vi "Dashboard Main.vi"() -> ()   [LabVIEW 2020]
uses:
  <vilib>/Utility/miscctls.llb/LVRowAndColumnTypeDef.ctl
  <vilib>/event_ctls.llb/eventvkey.ctl
  <vilib>/Rock Robotics/Network Tables/NT Read Numeric Array.vi
  <vilib>/Rock Robotics/WPI/Dashboard/WPI_DashboardLogging Global.vi
  <vilib>/Rock Robotics/Network Tables/NT Read Variant.vi
panel:
  out "DriveSensorData":T1
  out "NT Connection":bool
  in  "Camera Settings Right":T2={"Frame Rate"=30, "Compression"=30, "Size"=1, "DB Camera Config"=FALSE} {"Frame Rate" scale=1.0..30.0; "Compression" scale=100.0..-1.0; "Size" items=["640x480", "320x240", "160x120"]}
  in  "Camera Name Right":string(combo)="No Camera Selection"
  out "Camera Perf":string
  in  "Camera Settings":T2={"Frame Rate"=30, "Compression"=30, "Size"=1, "DB Camera Config"=FALSE} {"Frame Rate" scale=1.0..30.0; "Compression" scale=100.0..-1.0; "Size" items=["640x480", "320x240", "160x120"]}
  in  "TCP":refnum<k5>
  in  "Rec Mode":enum32{"Stop", "Record", "Playback"}(radio)
  out "Robot IP":string
  out "Image Message":string="Timeout in Camera Communications"
  in  "Dashboard Tab":T3(tab)
  out "Mode":T4(ring)=enum."Auto Disabled"
  out "Right Camera Perf":cluster{"Bandwidth (Mbps)":dbl, "FPS":dbl}
  in  "StartingPosition":dbl
  in  "AutoFileName (No .txt)":string
  in  "WaitAtStartOfAuto (Seconds)":dbl
  out "AutoFilesOnRobot":string[](array[string])
  out "Camera Image Right":T5(plugin-control)
  in  "DB/String 9":string
  in  "DB/String 8":string
  in  "DB/String 7":string
  in  "DB/String 6":string
  in  "DB/String 5":string
  in  "DB/String 4":string
  in  "DB/String 3":string
  in  "DB/String 2":string
  in  "DB/String 1":string
  in  "DB/String 0":string
  in  "DB/Slider 0":dbl(slide) scale=0.0..5.0
  in  "DB/Slider 1":dbl(slide) scale=0.0..5.0
  in  "DB/Slider 2":dbl(slide) scale=0.0..5.0
  in  "DB/Slider 3":dbl(slide) scale=0.0..5.0
  out "DB/LED 3":bool
  out "DB/LED 2":bool
  out "DB/LED 1":bool
  out "DB/LED 0":bool
  in  "DB/Button 3":bool
  in  "DB/Button 2":bool
  in  "DB/Button 1":bool
  in  "DB/Button 0":bool caption="New Name"
  in  "Test Slider":dbl(slide) scale=0.0..100.0 scale format="%#_3g"
  in  "On/Off":bool caption="Solenoid"
  in  "Test Name":u16(ring) items=["Select the test to run..."]
  in  "Test Tree":string(tree)
  in  "Motor":cluster{"Value":dbl, "Enable":bool} {"Value" scale=-1.0..1.0 scale format="%#_3g"}
  out "Progress":T6 {"Test Progress" scale=0.0..100.0}
  in  "Rev/Fwd":cluster{"Forward":bool, "Reverse":bool}
  in  "Test Ring":u16(ring) items=["Monochrome", "Color"]
  out "Cmd Status":string
  in  "Execute Command":bool
  in  "Command Params":string[][](table)
  in  "Command Selection":i32(listbox)
  in  "CheckList":i32(listbox)
  out "Tree":string(tree)
  out "Camera Image":T5(plugin-control)
  in  "Camera Name":string(combo)="No Camera Selection"
  # "HW"
  # "HW"
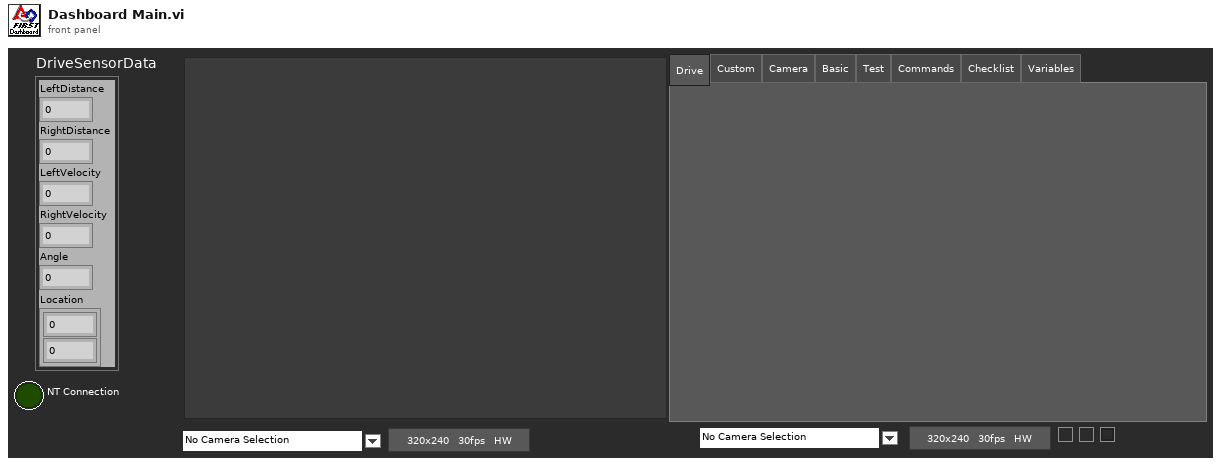
[diagram p1: front panel]
types:
  T1 = cluster{"LeftDistance":dbl, "RightDistance":dbl, "LeftVelocity":dbl, "RightVelocity":dbl, "Angle":dbl, "Location":cluster{dbl, dbl}}
  T2 = cluster{"Frame Rate":i32, "Compression":i32, "Size":u16, "DB Camera Config":bool}
  T3 = enum32{"Drive", "Custom", "Camera", "Basic", "Test", "Commands", "Checklist", "Variables"}
  T4 = enum8{"Tele-Op Disabled", "Tele-Op Enabled", "Auto Disabled", "Auto Enabled", "Test Disabled", "Test Enabled", "Disconnected", "No Code", "E-Stop"}
  T5 = typedef "IMAQ Image.ctl" = refnum<image>
  T6 = cluster{"Test Progress":u8, "Test Progress Text":string}
  T7 = cluster{"Save Path":path, "Interval (s)":dbl, "Keep":i32}
  T8 = enum32{"Drive", "Camera", "Basic", "Custom", "Test", "Commands", "Checklist", "Variables"}
  T9 = typedef "Image Type" = u32
  T10 = cluster{"IDs":cluster{"RPC field ID":u16, "Unique ID":u16}, "String":string}
  T11 = cluster{"Error Strings":string, "Disable Counts":cluster{u16, u16}, "Rail Faults":cluster{u16, u16, u16}, "Robot IP":string, "DB Mode":u8, "Event Info":cluster{"Name":string, "Type":u8, "Number":u16, "Replay":u8}}
  T12 = cluster{"Storage":cluster{"Disk Free":u64, "RAM Block":u32, "RAM free":u32}, "CPU Utilization":cluster{"CPU % ISR":sgl, "CPU % Time Crit":sgl, "CPU % Timed Str":sgl, "CPU % High":sgl, "CPU % Above":sgl, "CPU % Normal":sgl, "CPU % Low":sgl}, "CAN":cluster{"% Bus Utilization":sgl, "Bus Off Cnt":u32, "TX_FIFO Full Cnt":u32, "Receive Error Cnt":u8, "Transmit Error Cnt":u8}, "HID":cluster{"HID Outputs":u32, "Rumble Low":u16, "Rumble High":u16}[]}
  T13 = cluster{"Status bits":cluster{"Test Mode":bool, "Autonomous":bool, "Enabled":bool, "Code Start":bool, "Brownout":bool, "Reserved 2":bool, "Reserved 3":bool, "E-Stop":bool}, "Code Trace":cluster{"Disabled":bool, "TeleOp":bool, "Auto":bool, "Test":bool}, "Controller Type":enum16{"unknown", "cRIO", "roboRio"}, "Code?":enum16{"unknown", "noCode", "code"}, "Battery V":dbl}
  T14 = cluster{"Control Bits":cluster{"TestMode":bool, "Autonomous":bool, "Enabled":bool, "FMS Present":bool, bool, bool, bool, "E-Stop":bool}, "Team Station ":u8, "Countdown":sgl, "Joystick Values":cluster{"Axes":dbl[], "Buttons":bool[], "POVs":i16[]}[]}
  T15 = cluster{"Axes":dbl[], "Buttons":bool[], "POVs":i16[]}[]
  T16 = cluster{"Axes":dbl[], "Buttons":bool[], "POVs":i16[]}
  T17 = cluster{"Global Rectangle":i32[], "Contours":cluster{"Contour Type":u32, "ROI Type":u32, "Points":i32[]}[]}
  T18 = cluster{"Camera Name":string, string, "Saved DB Images Info":cluster{"Save Path":path, "Interval (s)":dbl, "Keep":i32}}
  T19 = cluster{"Camera Name Right":string, string, "Saved DB Images Info":cluster{"Save Path":path, "Interval (s)":dbl, "Keep":i32}}
  T20 = cluster{"Operation":enum16{"Update", "Clear"}, "Color Box":u32}[]
  T21 = typedef "eventvkey.ctl" = enum16{"ASCII", "Enter", "Return", "Shift", "Ctrl", "Alt", "Cmd", "Opt", "Caps", "NumLock", "Clear", "Break", "Up", "Down", "Left", "Right", "Insert", "Delete", "Home", "End", "PageUp", "PageDown", "Escape", "Help", "Pause", "ScrollLock", "F1", "F2", "F3", "F4", "F5", "F6", "F7", "F8", "F9", "F10", "F11", "F12", "F13", "F14", "F15", "F16", "F17", "F18", "F19", "F20", "F21", "F22", "F23", "F24", "Play", "VolumeUp", "VolumeDown", "Mute", "Two Byte Char"}
  T22 = cluster{"Image Size":bool, "Image Type":bool, "Pixel Value":bool, "ROI Information":bool, "Zoom Factor":bool}
  T23 = cluster{"Operation":enum16{"Update", "Clear"}, "Color Box":u32}
  T24 = typedef "LVRowAndColumnTypeDef.ctl" = cluster{"Row":i32, "Column":i32}
  T25 = cluster{"Shift":bool, "Ctrl":bool, "Alt":bool, "Cmd":bool, "Opt":bool}
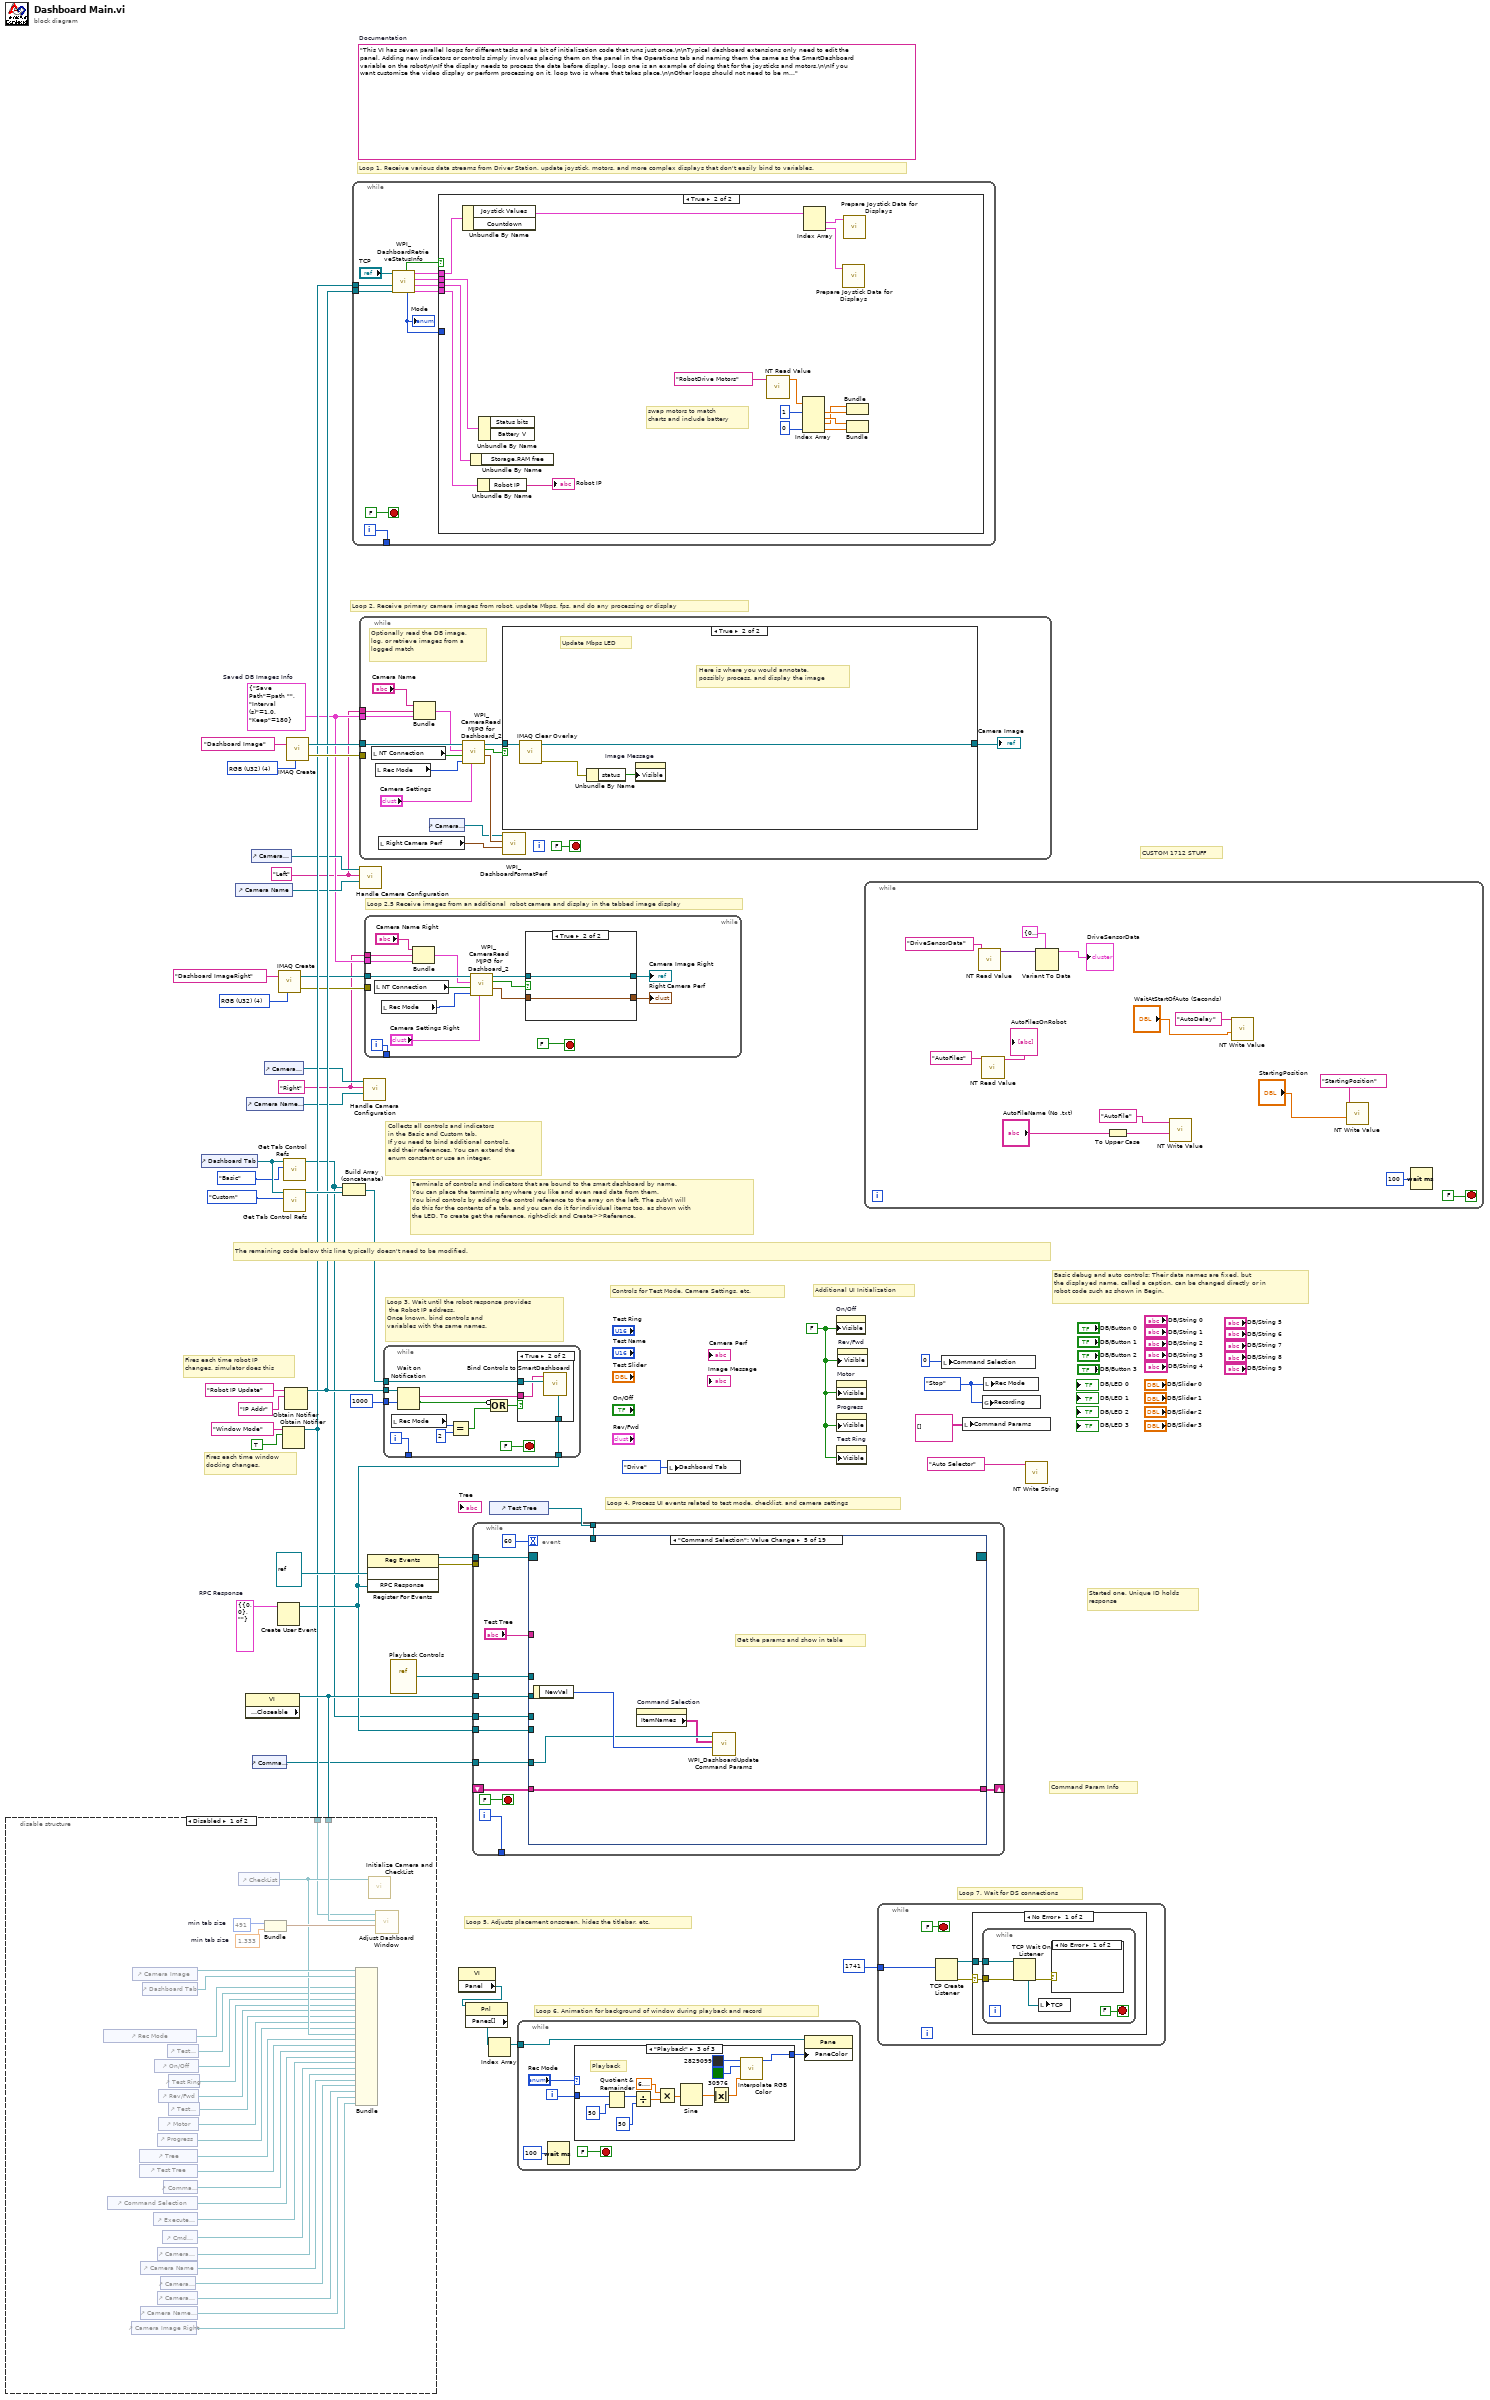
[diagram p0: block diagram]
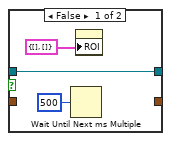
[diagram p3: hidden frame]
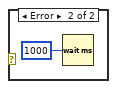
[diagram p4: hidden frame]
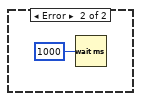
[diagram p5: hidden frame]
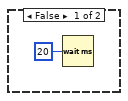
[diagram p6: hidden frame]
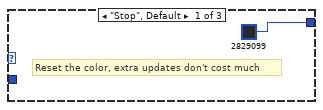
[diagram p7: hidden frame]
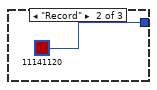
[diagram p8: hidden frame]
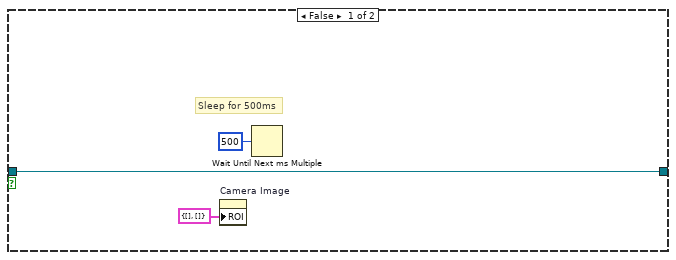
[diagram p10: hidden frame]
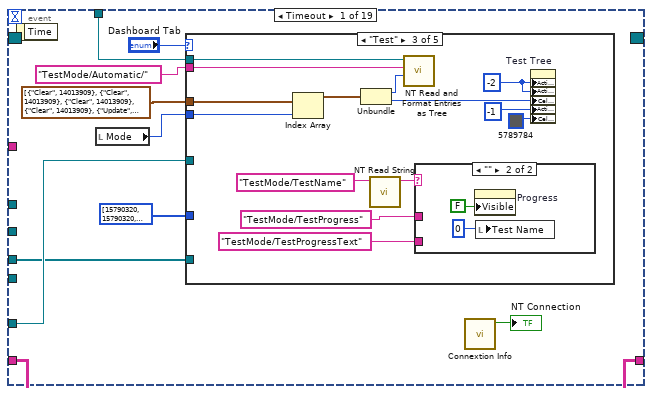
[diagram p11: hidden frame]
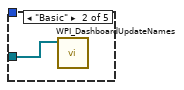
[diagram p13: hidden frame]
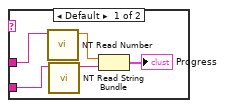
[diagram p14: hidden frame]
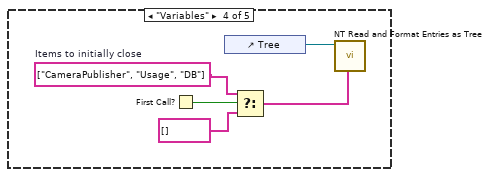
[diagram p15: hidden frame]
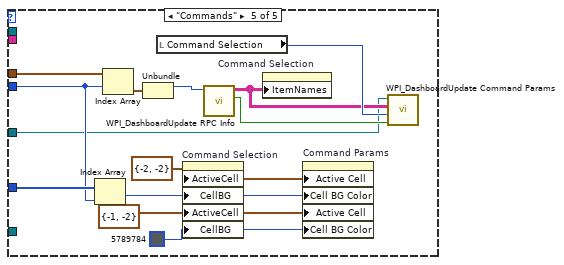
[diagram p16: hidden frame]
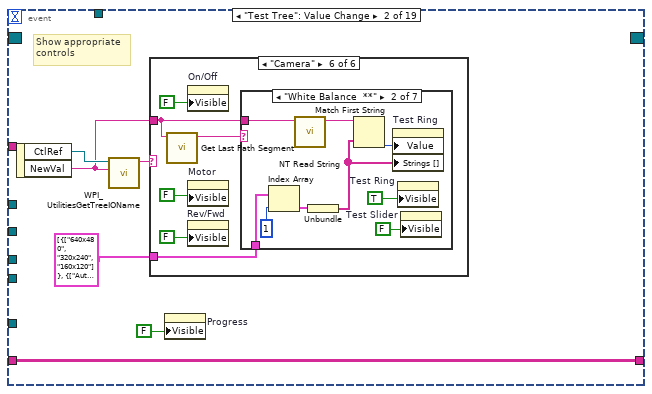
[diagram p17: hidden frame]
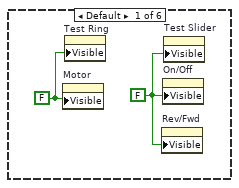
[diagram p18: hidden frame]
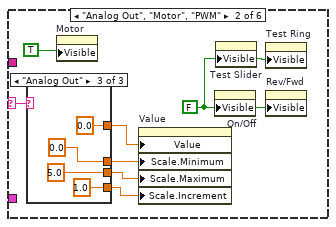
[diagram p19: hidden frame]
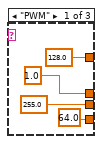
[diagram p20: hidden frame]
diagram:
  w4 = T7 {"Save Path"=path "", "Interval (s)"=1.0, "Keep"=180}  # Saved DB Images Info
  w3 = "Right"
  w2 = "Left"
  w11 = T9 4 items=["Grayscale (U8)", "Grayscale (I16)", "Grayscale (SGL)", "Complex (CSG)", "RGB (U32)", "HSL (U32)", "RGB (U64)"] ("Image Type")
  w21 = T10 {"IDs"={"RPC field ID"=0, "Unique ID"=0}, "String"=""}  # RPC Response
  w30 = enum32{"Stop", "Record", "Playback"}."Stop" ("Rec Mode")
  w25 = FALSE ("Visible")
  (unwired) "This VI has seven parallel loops for different tasks and a bit of initialization code that runs just once.\n\nTypical dashboard extensions only need to edit the panel. Adding new indicators or controls simply involves placing them on the panel in the Operations tab and naming them the same as the SmartDashboard variable on the robot\n\nIf the display needs to process the data before display, loop one is an example of doing that for the joysticks and motors.\n\nIf you want customize the video display or perform processing on it, loop two is where that takes place.\n\nOther loops should not need to be modified. They are pretty standard, and document the task they perform."  # Documentation
  w47 = T9 4 items=["Grayscale (U8)", "Grayscale (I16)", "Grayscale (SGL)", "Complex (CSG)", "RGB (U32)", "HSL (U32)", "RGB (U64)"] ("Image Type")
  # "CUSTOM 1712 STUFF"
  # "Loop 2.5 Receive images from an additional  robot camera and display in the tabbed image display"
  # "Command Param Info"
  # "Started one, Unique ID holds\nresponse"
  # "Loop 7. Wait for DS connections"
  # "Basic debug and auto controls: Their data names are fixed, but\nthe displayed name, called a caption, can be changed directly or in\nrobot code such as shown in Begin."
  # "Controls for Test Mode, Camera Settings, etc."
  # "Additional UI Initialization"
  # "Loop 6. Animation for background of window during playback and record"
  # "Fires each time robot IP\nchanges, simulator does this"
  # "Fires each time window\ndocking changes."
  # "Collects all controls and indicators\nin the Basic and Custom tab.\nIf you need to bind additional controls,\nadd their references. You can extend the\nenum constant or use an integer."
  # "The remaining code below this line typically doesn't need to be modified."
  # "Loop 4. Process UI events related to test mode, checklist, and camera settings"
  # "Terminals of controls and indicators that are bound to the smart dashboard by name.\nYou can place the terminals anywhere you like and even read data from them.\nYou bind controls by adding the control reference to the array on the left. The subVI will\ndo this for the contents of a tab, and you can do it for individual items too, as shown with\nthe LED. To create get the reference, right-click and Create>>Reference."
  # "Loop 3. Wait until the robot response provides\n the Robot IP address.\nOnce known, bind controls and\nvariables with the same names."
  # "Loop 5. Adjusts placement onscreen, hides the titlebar, etc."
  # "Loop 1. Receive various data streams from Driver Station, update joystick, motors, and more complex displays that don't easily bind to variables."
  # "Loop 2. Receive primary camera images from robot, update Mbps, fps, and do any processing or display"
  n1 = control-ref of="Dashboard Tab"() -> (w28:refnum<vi>)
  n2 = control-ref of="Camera Name"() -> (w15:refnum<vi>)
  n3 = property class="VI" props=["Front Panel.Closeable"]() -> (reference out=w29:refnum<vi>)  [unwired: 2 in, 2 out]
  n4 = control-ref of="Camera Name Right"() -> (w7:refnum<vi>)
  n5 = control-ref of="Camera Settings"() -> (w16:refnum<vi>)
  n6 = control-ref of="Command Params"() -> (w17:refnum<vi>)
  n7 = control-ref of="Camera Settings Right"() -> (w8:refnum<vi>)
  n8 = Create User Event(user event datatype=w21) -> (user event=w18:refnum<user-event>)  [unwired: 1 in, 1 out]
  n9 = call "IMAQ Create"("Image Name"="Dashboard ImageRight", "Image Type"=w11) -> ("New Image"=w10:T5, "error out"=w9:errorcluster)  [unwired: 2 in, 1 out]
  n10 = Obtain Notifier(name (unnamed)="Window Mode", notification data type=TRUE) -> (notifier out=w23:refnum<notifier>)  [unwired: 2 in, 2 out]
  n11 = disable-structure shown="Disabled" {
    disable-tunnel: w29 -> [w75 _]
    disable-tunnel: w23 -> [w58 _]
    frame Disabled {
      w72 = 491  # min tab size
      w71 = 1.333  # min tab size
      n12 = control-ref of="Rec Mode"() -> (w64:refnum<vi>)
      n13 = control-ref of="Command Selection"() -> (w55:refnum<vi>)
      n14 = control-ref of="Camera Image Right"() -> (w48:refnum<vi>)
      n15 = control-ref of="Camera Image"() -> (w74:refnum<vi>)
      n16 = control-ref of="Tree"() -> (w68:refnum<vi>)
      n17 = control-ref of="Test Tree"() -> (w67:refnum<vi>)
      n18 = control-ref of="Camera Name"() -> (w52:refnum<vi>)
      n19 = control-ref of="Camera Name Right"() -> (w49:refnum<vi>)
      n20 = control-ref of="Dashboard Tab"() -> (w73:refnum<vi>)
      n21 = control-ref of="Execute Command"() -> (w56:refnum<vi>)
      n22 = control-ref of="On/Off"() -> (w62:refnum<vi>)
      n23 = control-ref of="Progress"() -> (w59:refnum<vi>)
      n24 = control-ref of="Camera Settings"() -> (w53:refnum<vi>)
      n25 = control-ref of="Camera Settings Right"() -> (w50:refnum<vi>)
      n26 = control-ref of="Rev/Fwd"() -> (w60:refnum<vi>)
      n27 = control-ref of="Motor"() -> (w65:refnum<vi>)
      n28 = control-ref of="Camera Perf"() -> (w51:refnum<vi>)
      n29 = control-ref of="Cmd Status"() -> (w54:refnum<vi>)
      n30 = control-ref of="Command Params"() -> (w57:refnum<vi>)
      n31 = control-ref of="Test Slider"() -> (w63:refnum<vi>)
      n32 = control-ref of="Test Ring"() -> (w61:refnum<vi>)
      n33 = control-ref of="Test Name"() -> (w66:refnum<vi>)
      n34 = control-ref of="CheckList"() -> (w69:refnum<vi>)
      n35 = Bundle("min tab size"=w72, "min tab size"=w71) -> (w70:cluster{"min tab size":i32, "min tab size":dbl})  [unwired: 1 in]
      n36 = Bundle("Camera Image"=w74, "Dashboard Tab"=w73, "Rec Mode"=w64, "Test Slider"=w63, "On/Off"=w62, "Test Ring"=w61, "Rev/Fwd"=w60, "Test Name"=w66, "Motor"=w65, "Progress"=w59, "CheckList"=w69, "Tree"=w68, "Test Tree"=w67, "Command Params"=w57, "Command Selection"=w55, "Execute Command"=w56, "Cmd Status"=w54, "Camera Settings"=w53, "Camera Name"=w52, "Camera Perf"=w51, "Camera Settings Right"=w50, "Camera Name Right"=w49, "Camera Image Right"=w48) -> ()  [unwired: 2 in, 1 out]
      n37 = call "Initialize Camera and CheckList.vi"("ListBox in"=w69) -> ()  [unwired: 11 in]
      n38 = call "Adjust Dashboard Window.vi"("Size Constraints"=w70, "VI"=w75, "WIn Mode"=w58) -> ()  [unwired: 9 in]
    }
    frame Enabled {
    }
  }
  n39 = call <vilib>:"Get Tab Control Refs.vi"("Page Index"=T8."Basic" ("Dashboard Tab"), "TabControl in"=w28) -> ("ControlsOnPage"=w14:refnum<vi>[])  [unwired: 9 in]
  n40 = call <vilib>:"Get Tab Control Refs.vi"("Page Index"=T8."Custom" ("Dashboard Tab"), "TabControl in"=w28) -> ("ControlsOnPage"=w27:refnum<vi>[])  [unwired: 9 in]
  n41 = Obtain Notifier(name (unnamed)="Robot IP Update", notification data type="IP Addr" ("name (unnamed)")) -> (notifier out=w24:refnum<notifier>)  [unwired: 2 in, 2 out]
  n42 = call "IMAQ Create"("Image Name"="Dashboard Image", "Image Type"=w47) -> ("New Image"=w45:T5, "error out"=w44:errorcluster)  [unwired: 2 in, 1 out]
  n43 = Build Array (concatenate)(w14, w27) -> (w26:refnum<vi>[])
  n44 = while {
    tunnel: [w85] -> _
    tunnel: w24 -> [w79]
    tunnel: w23 -> [w76]
    i -> [w85]
    stop <- FALSE stop-if-true
    n45 = call <vilib>:"WPI_DashboardRetrieveStatusInfo.vi"("Binding Refnum"=w79, "Window Mode Notifier"=w76, "TCP Cnx"="TCP") -> ("Power and Errors"=w80:T11, "Robot Metrics"=w83:T12, "Status Info"=w84:T13, "Control Info"=w81:T14, "Robot Mode"=w78:T4, "Process?"=w82:bool)  [unwired: 3 in]
    "Mode" <- w78
    n46 = case shown="True" w82 {
      tunnel: w84 -> [_ w103]
      tunnel: w83 -> [_ w102]
      tunnel: w81 -> [_ w101]
      tunnel: w80 -> [_ w100]
      tunnel: w78 -> [_ _]
      frame False {
        n47 = Wait (ms)(milliseconds to wait=u32 20) -> ()  [unwired: 1 out]
      }
      frame True {
        # "swap motors to match\ncharts and include battery"
        n48 = Unbundle By Name(w101) -> ("Joystick Values"=w93:T15)  [unwired: 1 out]
        n49 = Unbundle By Name(w102) -> ()  [unwired: 1 out]
        n50 = Unbundle By Name(w100) -> ("Robot IP"=→"Robot IP":string)
        n51 = Unbundle By Name(w103) -> ()  [unwired: 2 out]
        n52 = call-poly <vilib>:"NT Read Value.vi"("Name"="RobotDrive Motors") -> ("Numeric Array"=w89:dbl[])  [unwired: 9 in, 1 out]
        n53 = Index Array(array=w89, index #1=1, index #4=0) -> (element #1=w95:dbl, element #2=w96:dbl, element #3=w94:dbl, element #4=w99:dbl)  [unwired: 2 in]
        n54 = Index Array(array=w93) -> (element #1=w92:T16, element #2=w91:T16)  [unwired: 2 in]
        n55 = call "Prepare Joystick Data for Displays.vi"("Joystick Values"=w91) -> ()  [unwired: 8 in, 3 out]
        n56 = call "Prepare Joystick Data for Displays.vi"("Joystick Values"=w92) -> ()  [unwired: 8 in, 3 out]
        n57 = Bundle("Numeric"=w94, "Numeric"=w95) -> ()  [unwired: 1 in, 1 out]
        n58 = Bundle("Numeric"=w96, "Numeric"=w99) -> ()  [unwired: 1 in, 1 out]
      }
    }
  }
  n59 = call "Handle Camera Configuration.vi"("CameraNameRef"=w15, "Display Name"=w2, "ClusterRef"=w16) -> ()  [unwired: 9 in]
  n60 = while {
    tunnel: w45 -> [w117]
    tunnel: w44 -> [_]
    tunnel: w4 -> [w110]
    tunnel: w2 -> [w107]
    stop <- FALSE stop-if-true
    # "Optionally read the DB image,\nlog, or retrieve images from a\nlogged match"
    n61 = local read "NT Connection"() -> (w111:bool)
    n62 = local read "Rec Mode"() -> (w114:enum32{"Stop", "Record", "Playback"})
    n63 = local read "Right Camera Perf"() -> (w105:cluster{"Bandwidth (Mbps)":dbl, "FPS":dbl})
    n64 = Bundle("Camera Name"="Camera Name", w107, "Saved DB Images Info"=w110) -> (w109:T18)  [unwired: 1 in]
    n65 = control-ref of="Camera Perf"() -> (w104:refnum<vi>)
    n66 = call <vilib>:"WPI_CameraRead MJPG for Dashboard_2.vi"("Camera Settings"="Camera Settings", "Rec Mode"=w114, "NT Connection"=w111, "Capture Info"=w109, "Image in"=w117) -> ("perf info"=w106:cluster{"Bandwidth (Mbps)":dbl, "fps":dbl}, "Active"=w115:bool, "Image\\ out"=w116:T5)  [unwired: 4 in]
    n67 = case shown="True" w115 {
      tunnel: w116 -> [w120 w123]
      tunnel: [w120 w122] -> w112
      frame False {
        # "Sleep for 500ms"
        n68 = property on="Camera Image" class="ImageControl"("ROI"=T17 {"Global Rectangle"=[], "Contours"=[]}) -> ()  [unwired: 2 in, 2 out]
        n69 = Wait Until Next ms Multiple(millisecond multiple=u32 500) -> ()  [unwired: 1 out]
      }
      frame True {
        # "Here is where you would annotate,\npossibly process, and display the image"
        # "Update Mbps LED"
        n70 = call "IMAQ Clear Overlay"("Image"=w123) -> ("error out"=w124:errorcluster, "Image Out"=w122:T5)  [unwired: 2 in, 7 out]
        n71 = Unbundle By Name(w124) -> ("status"=w125:bool)
        n72 = property on="Image Message" class="Str"("Visible"=w125) -> ()  [unwired: 2 in, 2 out]
      }
    }
    "Camera Image" <- w112
    n73 = call <vilib>:"WPI_DashboardFormatPerf.vi"("Right Camera Perf"=w105, "Performance"=w106, "String in"=w104) -> ()  [unwired: 9 in]
  }
  n74 = call "Handle Camera Configuration.vi"("CameraNameRef"=w7, "Display Name"=w3, "ClusterRef"=w8) -> ()  [unwired: 9 in]
  n75 = while {
    tunnel: w10 -> [w140]
    tunnel: w9 -> [_]
    tunnel: [w135] -> _
    tunnel: w4 -> [w131]
    tunnel: w3 -> [w128]
    i -> [w135]
    stop <- FALSE stop-if-true
    n76 = local read "NT Connection"() -> (w132:bool)
    n77 = local read "Rec Mode"() -> (w139:enum32{"Stop", "Record", "Playback"})
    n78 = Bundle("Camera Name Right"="Camera Name Right", w128, "Saved DB Images Info"=w131) -> (w130:T19)  [unwired: 1 in]
    n79 = call <vilib>:"WPI_CameraRead MJPG for Dashboard_2.vi"("Camera Settings"="Camera Settings Right", "Rec Mode"=w139, "NT Connection"=w132, "Capture Info"=w130, "Image in"=w140) -> ("perf info"=w126:cluster{"Bandwidth (Mbps)":dbl, "fps":dbl}, "Active"=w134:bool, "Image\\ out"=w137:T5)  [unwired: 4 in]
    n80 = case shown="True" w134 {
      tunnel: w137 -> [w142 w145]
      tunnel: [w142 w145] -> w133
      tunnel: [_ w144] -> w127
      tunnel: w126 -> [_ w144]
      frame False {
        n81 = Wait Until Next ms Multiple(millisecond multiple=u32 500) -> ()  [unwired: 1 out]
        n82 = property on="Camera Image Right" class="ImageControl"("ROI"=T17 {"Global Rectangle"=[], "Contours"=[]}) -> ()  [unwired: 2 in, 2 out]
      }
      frame True {
      }
    }
    "Camera Image Right" <- w133
    "Right Camera Perf" <- w127
  }
  n83 = register-events(refnum<vi> refnum, w18) -> (reference out=w34:refnum<event-registration>, error out=w33:errorcluster)  [unwired: 2 in]
  n84 = while {
    tunnel: w26 -> [w157]
    tunnel: w24 -> [w155]
    tunnel: [w153] -> _
    tunnel: u32 1000 ("milliseconds to wait") -> [w152]
    tunnel: w18 -> [w146]
    i -> [w153]
    stop <- FALSE stop-if-true
    n85 = local read "Rec Mode"() -> (w148:enum32{"Stop", "Record", "Playback"})
    n86 = Wait on Notification(notifier=w155, timeout in ms (-1)=w152) -> (notification=w154:string, timed out?=w150:bool)  [unwired: 2 in, 2 out]
    n87 = Equal?(x=w148, y=u16 2 ("Rec Mode")) -> (x = y?=w149:bool)
    n88 = Compound Arithmetic op=OR(invert w150, w149) -> (w151:bool)
    n89 = case shown="True" w151 {
      tunnel: w157 -> [_ w160]
      tunnel: w154 -> [_ w159]
      tunnel: w146 -> [_ w158]
      frame False {
      }
      frame True {
        n90 = call <vilib>:"Bind Controls to SmartDashboard.vi"("RPC ref"=w158, "Bound Control Refs"=w160, "Server IP Address"=w159) -> ()  [unwired: 9 in]
      }
    }
  }
  n91 = vi-ref "Playback Controls.vi"() -> (w35:refnum<vi>)
  n92 = property class="VI"() -> ("Panel"=w37:refnum<vi>)  [unwired: 2 in, 2 out]
  n93 = property class="Pnl"(reference=w37) -> ("Panes[]"=w38:refnum<vi>[])  [unwired: 1 in, 2 out]
  n94 = Index Array(array=w38) -> (element=w36:refnum<vi>)  [unwired: 1 in]
  n95 = control-ref of="Test Tree"() -> (w39:refnum<vi>)
  n96 = while {
    tunnel: [w170] -> _
    tunnel: w39 -> [w169]
    tunnel: w35 -> [w168]
    tunnel: w34 -> [w167]
    tunnel: w33 -> [_]
    tunnel: w29 -> [w166]
    tunnel: w18 -> [w165]
    tunnel: w17 -> [w164]
    shift-right: [w163] -> _
    shift-left: _ -> [w162]
    tunnel: w14 -> [w161]
    i -> [w170]
    stop <- FALSE stop-if-true
    n97 = event shown="[4] \"Command Selection\": Value Change" {
      selector: w167 -> [_ _ _ _ _ _ _ _ _ _ _ _ _ _ _ _ _ _ _]
      dyn-events: [_ _ _ _ _ _ _ _ _ _ _ _ _ _ w424 _ _ _ _] -> _
      timeout: u32 60 ("milliseconds to wait") -> [_ _ _ _ _ _ _ _ _ _ _ _ _ _ _ _ _ _ _]
      tunnel: w169 -> [w182 _ _ _ _ _ _ _ _ _ _ _ _ _ _ _ _ _ _]
      tunnel: "Test Tree" -> [_ _ _ _ _ _ _ _ _ w391 w399 w401 w405 w413 _ _ _ _ _]
      tunnel: w168 -> [_ _ _ _ _ _ _ _ _ _ _ _ _ _ w426 _ w444 _ _]
      tunnel: w166 -> [_ _ _ _ _ _ _ _ _ _ _ _ _ _ w422 _ _ _ _]
      tunnel: w165 -> [_ _ _ _ _ _ _ _ _ _ _ _ _ _ w420 _ _ _ _]
      tunnel: w164 -> [w177 _ _ _ w342 _ _ _ _ _ _ _ _ _ _ _ _ _ _]
      tunnel: [w176 w225 w327 w332 w340 w349 w359 w366 w378 w390 w397 w400 w404 w412 w419 w439 w441 w445 w458] -> w163
      tunnel: w162 -> [w176 w225 w327 w332 w340 _ _ w366 w378 w390 w397 w400 w404 w412 w419 w439 w441 w445 w458]
      tunnel: w161 -> [w174 _ _ _ _ _ _ _ _ _ _ _ _ _ _ _ _ _ _]
      event Timeout {
        n98 = event-data() -> ()  [unwired: 1 in, 1 out]
        n99 = local read "Mode"() -> (w179:T4)
        n100 = case shown="\"Test\"" "Dashboard Tab" {
          tunnel: w182 -> [_ _ w198 _ _]
          tunnel: "TestMode/Automatic/" ("Name Pattern") -> [_ _ w197 _ _]
          tunnel: T20 [{"Operation"=enum."Clear", "Color Box"=14013909}, {"Operation"=enum."Clear", "Color Box"=14013909}, {"Operation"=enum."Clear", "Color Box"=14013909}, {"Operation"=enum."Clear", "Color Box"=14013909}, {"Operation"=enum."Update", "Color Box"=14013909}, {"Operation"=enum."Update", "Color Box"=16777215}, {"Operation"=enum."Clear", "Color Box"=14013909}, {"Operation"=enum."Clear", "Color Box"=14013909}, {"Operation"=enum."Clear", "Color Box"=14013909}] -> [_ _ w190 _ w218]
          tunnel: w179 -> [_ _ w189 _ w217]
          tunnel: u32[] [15790320, 15790320, 15790320, 15790320, 16777215, 16777215, 15790320, 15790320, 15790320] -> [_ _ _ _ w223]
          tunnel: w177 -> [_ _ _ _ w211]
          tunnel: w174 -> [_ w184 _ _ _]
          frame "Custom", Default {
          }
          frame "Basic" {
            n101 = call <vilib>:"WPI_DashboardUpdateNames.vi"("Controls on Tab"=w184) -> ()  [unwired: 11 in]
          }
          frame "Test" {
            w196 = -2 ("Active Item:Row Number")
            n102 = Index Array(array=w190, index=w189) -> (element=w191:T23)
            n103 = Unbundle(w191) -> ("Operation"=w192:enum16{"Update", "Clear"}, "Color Box"=w193:u32)
            n104 = call <vilib>:"NT Read String.vi"("Name"="TestMode/TestName") -> ("String"=w187:string)  [unwired: 9 in, 1 out]
            n105 = call <vilib>:"NT Read and Format Entries as Tree.vi"("Operation"=w192, "Name Pattern"=w197, "Tree Refnum"=w198) -> ()  [unwired: 7 in, 2 out]
            n106 = case shown="\"\"" w187 {
              tunnel: "TestMode/TestProgress" ("Name") -> [w200 _]
              tunnel: "TestMode/TestProgressText" ("Name") -> [w199 _]
              frame Default {
                n107 = call <vilib>:"NT Read Number.vi"("Name"=w200) -> ("Numeric"=w201:dbl)  [unwired: 9 in, 1 out]
                n108 = call <vilib>:"NT Read String.vi"("Name"=w199) -> ("String"=w202:string)  [unwired: 9 in, 1 out]
                n109 = Bundle("Numeric"=w201, "String"=w202) -> (→"Progress":cluster{"Numeric":dbl, "String":string})  [unwired: 1 in]
              }
              frame "" {
                n110 = property on="Progress" class="Clust (strict)"("Visible"=FALSE) -> ()  [unwired: 2 in, 2 out]
                n111 = local write "Test Name"(u16 0) -> ()
              }
            }
            n112 = property on="Test Tree" class="Tree (strict)"("Active Item Row Number"=w196, "ActiveColNum"=w196, "CellBG"=w193, "Active Item Row Number"=-1 ("Active Item:Row Number"), "CellBG"=u32 5789784 ("Color Box")) -> ()  [unwired: 2 in, 2 out]
          }
          frame "Variables" {
            w208 = string[] ["CameraPublisher", "Usage", "DB"]  # Items to initially close
            n113 = First Call?() -> (First Call?: T/F=w209:bool)
            n114 = control-ref of="Tree"() -> (w210:refnum<vi>)
            n115 = Select(t=w208, s=w209, f=string[] []) -> (s? t:f=w206:string[])
            n116 = call <vilib>:"NT Read and Format Entries as Tree.vi"("Tags to  Close"=w206, "Tree Refnum"=w210) -> ()  [unwired: 8 in, 2 out]
          }
          frame "Commands" {
            w219 = u32 5789784 ("Color Box")
            w220 = T24 {"Row"=-1, "Column"=-2} ("Active Cell:Active Cell")
            w222 = T24 {"Row"=-2, "Column"=-2} ("Active Cell:Active Cell")
            n117 = Index Array(array=w223, index=w217) -> (element=w221:u32)
            n118 = Index Array(array=w218, index=w217) -> (element=w216:T23)
            n119 = Unbundle(w216) -> ("Operation"=w215:enum16{"Update", "Clear"})  [unwired: 1 out]
            n120 = local read "Command Selection"() -> (w214:i32)
            n121 = property on="Command Selection" class="MCListbox (strict)"("ActiveCell"=w222, "CellBG"=w221, "ActiveCell"=w220, "CellBG"=w219) -> ()  [unwired: 2 in, 2 out]
            n122 = call <vilib>:"WPI_DashboardUpdate RPC Info.vi"("Operation"=w215) -> ("update"=w213:bool, "commands"=w212:string[][])  [unwired: 9 in]
            n123 = property on="Command Selection" class="MCListbox (strict)"("ItemNames"=w212) -> ()  [unwired: 2 in, 2 out]
            n124 = property on="Command Params" class="Tbl (strict)"("Active Cell"=w222, "Cell BG Color"=w221, "Active Cell"=w220, "Cell BG Color"=w219) -> ()  [unwired: 2 in, 2 out]
            n125 = call <vilib>:"WPI_DashboardUpdate Command Params.vi"("Update"=w213, "NewVal"=w214, "Commands"=w212, "Param Tbl"=w211) -> ()  [unwired: 7 in, 1 out]
          }
        }
        n126 = call <vilib>:"Connextion Info.vi"() -> ("Connected"=→"NT Connection":bool)  [unwired: 10 in, 1 out]
      }
      event "Test Tree": Value Change {
        # "Show appropriate\ncontrols"
        n127 = event-data() -> ("CtlRef"=w228:refnum<vi>, "NewVal"=w226:string)  [unwired: 1 in]
        n128 = call <vilib>:"WPI_UtilitiesGetTreeIOName.vi"("NewVal"=w226, "TreeControl in"=w228) -> ("I/O Name"=w229:string)  [unwired: 9 in]
        n129 = case shown="\"Camera\"" w229 {
          selector: w229 -> [_ w236 _ w258 w267 _]
          tunnel: w226 -> [_ _ w255 w257 _ w274]
          tunnel: cluster{string[]}[] [{["640x480", "320x240", "160x120"]}, {["Auto", "Fixed indoor", "Fixed outdoor 1", "Fixed outdoor 2", "Fixed fluorescent 1", "Fixed fluorescent 2", "Hold current"]}, {["Auto", "Flicker-free 50 Hz", "Flicker-free 60 Hz", "Hold current"]}, {["None", "Prioritize frame rate", "Prioritize image quality"]}, {["Monochrome", "Color"]}] -> [_ _ _ _ _ w273]
          frame Default {
            w231 = FALSE ("Visible")
            w230 = FALSE ("Visible")
            n130 = property on="Motor" class="Clust (strict)"("Visible"=w230) -> ()  [unwired: 2 in, 2 out]
            n131 = property on="Test Ring" class="Ring (strict)"("Visible"=w230) -> ()  [unwired: 2 in, 2 out]
            n132 = property on="Rev/Fwd" class="Clust (strict)"("Visible"=w231) -> ()  [unwired: 2 in, 2 out]
            n133 = property on="On/Off" class="Bool (strict)"("Visible"=w231) -> ()  [unwired: 2 in, 2 out]
            n134 = property on="Test Slider" class="Slide (strict)"("Visible"=w231) -> ()  [unwired: 2 in, 2 out]
          }
          frame "Analog Out", "Motor", "PWM" {
            w237 = FALSE ("Visible")
            n135 = case shown="\"Analog Out\"" w236 {
              tunnel: [1.0 ("Value") -1.0 ("Value") 0.0 ("Value")] -> w235
              tunnel: [255.0 ("Value") 1.0 ("Value") 5.0 ("Value")] -> w234
              tunnel: [128.0 ("Value") 0.0 ("Value") 0.0 ("Value")] -> w233
              tunnel: [64.0 ("Value") 0.5 ("Value") 1.0 ("Value")] -> w232
              frame "PWM" {
              }
              frame "Motor", Default {
              }
              frame "Analog Out" {
              }
            }
            n136 = property on="Motor" class="Clust (strict)"("Visible"=TRUE) -> ()  [unwired: 2 in, 2 out]
            n137 = property on="Value" class="Slide (strict)"("Value"=w233, "Scale.Minimum"=w235, "Scale.Maximum"=w234, "Scale.Increment"=w232) -> ()  [unwired: 2 in, 2 out]
            n138 = property on="On/Off" class="Bool (strict)"("Visible"=w237) -> ()  [unwired: 2 in, 2 out]
            n139 = property on="Test Slider" class="Slide (strict)"("Visible"=w237) -> ()  [unwired: 2 in, 2 out]
            n140 = property on="Test Ring" class="Ring (strict)"("Visible"=w237) -> ()  [unwired: 2 in, 2 out]
            n141 = property on="Rev/Fwd" class="Clust (strict)"("Visible"=w237) -> ()  [unwired: 2 in, 2 out]
          }
          frame "Servo" {
            w253 = FALSE ("Visible")
            n142 = call <vilib>:"NT Read Number.vi"("Name"=w255) -> ("Numeric"=w254:dbl)  [unwired: 9 in, 1 out]
            n143 = property on="Test Slider" class="Slide (strict)"("Visible"=TRUE, "Scale.Maximum"=170.0 ("Scale.Range:Maximum")) -> ()  [unwired: 2 in, 2 out]
            n144 = local write "Test Slider"(w254) -> ()
            n145 = property on="Motor" class="Clust (strict)"("Visible"=w253) -> ()  [unwired: 2 in, 2 out]
            n146 = property on="Rev/Fwd" class="Clust (strict)"("Visible"=w253) -> ()  [unwired: 2 in, 2 out]
            n147 = property on="On/Off" class="Bool (strict)"("Visible"=w253) -> ()  [unwired: 2 in, 2 out]
            n148 = property on="Test Ring" class="Ring (strict)"("Visible"=w253) -> ()  [unwired: 2 in, 2 out]
          }
          frame "Relay", "Solenoid" {
            w256 = FALSE ("Visible")
            n149 = property on="Motor" class="Clust (strict)"("Visible"=w256) -> ()  [unwired: 2 in, 2 out]
            n150 = property on="Test Slider" class="Slide (strict)"("Visible"=w256) -> ()  [unwired: 2 in, 2 out]
            n151 = Search and Replace String(input string=w257, search string="/Value  **", replace string="/Direction") -> (result string=w263:string)  [unwired: 5 in, 3 out]
            n152 = property on="Test Ring" class="Ring (strict)"("Visible"=w256) -> ()  [unwired: 2 in, 2 out]
            n153 = call <vilib>:"NT Read String.vi"("Name"=w263) -> ("String"=w261:string)  [unwired: 9 in, 1 out]
            n154 = Equal?(x="Both directions", y=w261) -> (x = y?=w259:bool)
            n155 = Not(x=w259) -> (.not. x?=w260:bool)
            n156 = property on="Rev/Fwd" class="Clust (strict)"("Visible"=w259) -> ()  [unwired: 2 in, 2 out]
            n157 = property on="On/Off" class="Bool (strict)"("Visible"=w260, "Caption.Text"=w258) -> ()  [unwired: 2 in, 2 out]
          }
          frame "Compressor", "Digital Out" {
            w266 = FALSE ("Visible")
            # "Get direction and finish"
            n158 = property on="Motor" class="Clust (strict)"("Visible"=w266) -> ()  [unwired: 2 in, 2 out]
            n159 = property on="Test Slider" class="Slide (strict)"("Visible"=w266) -> ()  [unwired: 2 in, 2 out]
            n160 = property on="Test Ring" class="Ring (strict)"("Visible"=w266) -> ()  [unwired: 2 in, 2 out]
            n161 = property on="On/Off" class="Bool (strict)"("Visible"=TRUE, "Caption.Text"=w267) -> ()  [unwired: 2 in, 2 out]
            n162 = property on="Rev/Fwd" class="Clust (strict)"("Visible"=FALSE) -> ()  [unwired: 2 in, 2 out]
          }
          frame "Camera" {
            n163 = call <vilib>:"Get Last Path Segment.vi"("String in"=w274) -> ("String out"=w275:string)  [unwired: 10 in]
            n164 = property on="On/Off" class="Bool (strict)"("Visible"=FALSE) -> ()  [unwired: 2 in, 2 out]
            n165 = property on="Motor" class="Clust (strict)"("Visible"=FALSE) -> ()  [unwired: 2 in, 2 out]
            n166 = property on="Rev/Fwd" class="Clust (strict)"("Visible"=FALSE) -> ()  [unwired: 2 in, 2 out]
            n167 = case shown="\"White Balance  **\"" w275 {
              tunnel: w274 -> [w281 w290 w299 w308 w317 _ w323]
              tunnel: w273 -> [w279 w287 w296 w305 w314 _ _]
              frame "Size  **" {
                n168 = Index Array(array=w279) -> (element=w278:cluster{string[]})  [unwired: 1 in]
                n169 = call <vilib>:"NT Read String.vi"("Name"=w281) -> ("String"=w280:string)  [unwired: 9 in, 1 out]
                n170 = Unbundle(w278) -> (w276:string[])
                n171 = Match First String(2:w276, 3:w280) -> (0:w277:i32)  [unwired: 1 out]
                n172 = property on="Test Ring" class="Ring (strict)"("Value"=w277, "Strings []"=w276) -> ()  [unwired: 2 in, 2 out]
                n173 = property on="Test Ring" class="Ring (strict)"("Visible"=TRUE) -> ()  [unwired: 2 in, 2 out]
                n174 = property on="Test Slider" class="Slide (strict)"("Visible"=FALSE) -> ()  [unwired: 2 in, 2 out]
              }
              frame "White Balance  **" {
                n175 = Index Array(array=w287, index=1) -> (element=w288:cluster{string[]})
                n176 = call <vilib>:"NT Read String.vi"("Name"=w290) -> ("String"=w289:string)  [unwired: 9 in, 1 out]
                n177 = Unbundle(w288) -> (w285:string[])
                n178 = Match First String(2:w285, 3:w289) -> (0:w284:i32)  [unwired: 1 out]
                n179 = property on="Test Ring" class="Ring (strict)"("Value"=w284, "Strings []"=w285) -> ()  [unwired: 2 in, 2 out]
                n180 = property on="Test Ring" class="Ring (strict)"("Visible"=TRUE) -> ()  [unwired: 2 in, 2 out]
                n181 = property on="Test Slider" class="Slide (strict)"("Visible"=FALSE) -> ()  [unwired: 2 in, 2 out]
              }
              frame "Exposure  **" {
                n182 = Index Array(array=w296, index=2) -> (element=w297:cluster{string[]})
                n183 = call <vilib>:"NT Read String.vi"("Name"=w299) -> ("String"=w298:string)  [unwired: 9 in, 1 out]
                n184 = Unbundle(w297) -> (w293:string[])
                n185 = Match First String(2:w293, 3:w298) -> (0:w294:i32)  [unwired: 1 out]
                n186 = property on="Test Ring" class="Ring (strict)"("Value"=w294, "Strings []"=w293) -> ()  [unwired: 2 in, 2 out]
                n187 = property on="Test Ring" class="Ring (strict)"("Visible"=TRUE) -> ()  [unwired: 2 in, 2 out]
                n188 = property on="Test Slider" class="Slide (strict)"("Visible"=FALSE) -> ()  [unwired: 2 in, 2 out]
              }
              frame "Exposure Priority  **" {
                n189 = Index Array(array=w305, index=3) -> (element=w306:cluster{string[]})
                n190 = call <vilib>:"NT Read String.vi"("Name"=w308) -> ("String"=w307:string)  [unwired: 9 in, 1 out]
                n191 = Unbundle(w306) -> (w302:string[])
                n192 = Match First String(2:w302, 3:w307) -> (0:w303:i32)  [unwired: 1 out]
                n193 = property on="Test Ring" class="Ring (strict)"("Value"=w303, "Strings []"=w302) -> ()  [unwired: 2 in, 2 out]
                n194 = property on="Test Ring" class="Ring (strict)"("Visible"=TRUE) -> ()  [unwired: 2 in, 2 out]
                n195 = property on="Test Slider" class="Slide (strict)"("Visible"=FALSE) -> ()  [unwired: 2 in, 2 out]
              }
              frame "Color Enable  **" {
                n196 = Index Array(array=w314, index=4) -> (element=w315:cluster{string[]})
                n197 = call <vilib>:"NT Read String.vi"("Name"=w317) -> ("String"=w316:string)  [unwired: 9 in, 1 out]
                n198 = Unbundle(w315) -> (w311:string[])
                n199 = Match First String(2:w311, 3:w316) -> (0:w312:i32)  [unwired: 1 out]
                n200 = property on="Test Ring" class="Ring (strict)"("Value"=w312, "Strings []"=w311) -> ()  [unwired: 2 in, 2 out]
                n201 = property on="Test Ring" class="Ring (strict)"("Visible"=TRUE) -> ()  [unwired: 2 in, 2 out]
                n202 = property on="Test Slider" class="Slide (strict)"("Visible"=FALSE) -> ()  [unwired: 2 in, 2 out]
              }
              frame Default {
                n203 = property on="Test Ring" class="Ring (strict)"("Visible"=FALSE) -> ()  [unwired: 2 in, 2 out]
                n204 = property on="Test Slider" class="Slide (strict)"("Visible"=FALSE) -> ()  [unwired: 2 in, 2 out]
              }
              frame "Brightness  **", "Color Level  **", "Compression  **", "FPS  **", "Sharpness  **" {
                n205 = call <vilib>:"NT Read Number.vi"("Name"=w323) -> ("Numeric"=w322:dbl)  [unwired: 9 in, 1 out]
                n206 = local write "Test Slider"(w322) -> ()
                n207 = property on="Test Slider" class="Slide (strict)"("Visible"=TRUE, "Scale.Maximum"=100.0 ("Scale.Range:Maximum")) -> ()  [unwired: 2 in, 2 out]
                n208 = property on="Test Ring" class="Ring (strict)"("Visible"=FALSE) -> ()  [unwired: 2 in, 2 out]
              }
            }
          }
        }
        n209 = property on="Progress" class="Clust (strict)"("Visible"=FALSE) -> ()  [unwired: 2 in, 2 out]
      }
      event "Test Name": Mouse Enter {
        # "Populate the ring with the list of tests"
        n210 = event-data() -> ()  [unwired: 1 in, 1 out]
        n211 = call <vilib>:"NT Read String Array.vi"("Name"="TestMode/TestList") -> ("String Array"=w331:string[])  [unwired: 9 in, 1 out]
        n212 = Build Array (concatenate)("Select the test to run...", w331) -> (w330:string[])
        n213 = property on="Test Name" class="Ring (strict)"("Strings []"=w330) -> ()  [unwired: 2 in, 2 out]
      }
      event "Test Name": Value Change {
        w333 = FALSE ("Visible")
        # "Tell the robot the test name to run"
        n214 = event-data() -> ("NewVal"=w337:u16)  [unwired: 1 in]
        n215 = property on="Test Name" class="Ring (strict)"() -> ("Strings []"=w338:string[])  [unwired: 2 in, 2 out]
        n216 = local write "Progress"(T6 {"Test Progress"=0, "Test Progress Text"=""} ("Progress")) -> ()
        n217 = Index Array(array=w338, index=w337) -> (element=w336:string)
        n218 = call <vilib>:"NT Write String.vi"("String"=w336, "Name"="TestMode/TestName") -> ()  [unwired: 9 in, 1 out]
        n219 = property on="Progress" class="Clust (strict)"("Visible"=TRUE) -> ()  [unwired: 2 in, 2 out]
        n220 = property on="Motor" class="Clust (strict)"("Visible"=w333) -> ()  [unwired: 2 in, 2 out]
        n221 = property on="Test Slider" class="Slide (strict)"("Visible"=w333) -> ()  [unwired: 2 in, 2 out]
        n222 = property on="On/Off" class="Bool (strict)"("Visible"=w333) -> ()  [unwired: 2 in, 2 out]
        n223 = property on="Rev/Fwd" class="Clust (strict)"("Visible"=w333) -> ()  [unwired: 2 in, 2 out]
        n224 = property on="Test Ring" class="Ring (strict)"("Visible"=w333) -> ()  [unwired: 2 in, 2 out]
      }
      event "Command Selection": Value Change {
        # "Get the params and show in table"
        n225 = event-data() -> ("NewVal"=w343:i32)  [unwired: 1 in]
        n226 = property on="Command Selection" class="MCListbox (strict)"() -> ("ItemNames"=w341:string[][])  [unwired: 2 in, 2 out]
        n227 = call <vilib>:"WPI_DashboardUpdate Command Params.vi"("NewVal"=w343, "Commands"=w341, "Param Tbl"=w342) -> ()  [unwired: 8 in, 1 out]
      }
      event "Execute Command": Value Change {
        # "Started one, Unique ID holds\nresponse"
        n228 = event-data() -> ()  [unwired: 1 in, 1 out]
        n229 = property on="Command Selection" class="MCListbox (strict)"() -> ("ItemNames"=w354:string[][])  [unwired: 2 in, 2 out]
        n230 = Index Array(array=w354, index (row)="Command Selection", index (col)=0) -> (element=w352:string)
        n231 = call <vilib>:"Invoke Commands.vi"("Command Params"="Command Params", "Function Name"=w352) -> ("Params"=w348:u8, "Started"=w347:bool)  [unwired: 7 in, 1 out]
        n232 = Array Subset(array="Command Params", length (row)=w348) -> (w349:string[][])  [unwired: 3 in]
        n233 = Select(t="Executing" ("Cmd Status"), s=w347, f="" ("Cmd Status")) -> (s? t:f=→"Cmd Status":string)
      }
      event "Command Selection": Double Click {
        n234 = event-data() -> ("Row"=w362:i32)  [unwired: 1 in]
        n235 = property on="Command Selection" class="MCListbox (strict)"() -> ("ItemNames"=w365:string[][])  [unwired: 2 in, 2 out]
        n236 = local read "Command Params"() -> (w361:string[][])
        n237 = Index Array(array=w365, index (row)=w362, index (col)=0) -> (element=w363:string)
        n238 = call <vilib>:"Invoke Commands.vi"("Command Params"=w361, "Function Name"=w363) -> ("Params"=w360:u8, "Started"=w355:bool)  [unwired: 7 in, 1 out]
        n239 = Array Subset(array=w361, length (row)=w360) -> (w359:string[][])  [unwired: 3 in]
        n240 = Select(t="Executing" ("Cmd Status"), s=w355, f="" ("Cmd Status")) -> (s? t:f=w356:string)
        n241 = local write "Cmd Status"(w356) -> ()
      }
      event "CheckList": Double Click {
        # "Shift clears all"
        # "Update symbols on the listbox"
        n242 = event-data() -> ("PlatMods.Shift"=w367:bool, "Row"=w369:i32)  [unwired: 1 in]
        n243 = case shown="True" w367 {
          tunnel: w369 -> [w373 _]
          tunnel: 1 -> [w372 _]
          frame False {
            n244 = property on="CheckList" class="LstBox (strict)"() -> ("Item Symbols"=w371:i32[])  [unwired: 2 in, 2 out]
            n245 = Replace Array Subset(array=w371, new element=w372, index=w373) -> (w370:i32[])
            n246 = property on="CheckList" class="LstBox (strict)"("Item Symbols"=w370) -> ()  [unwired: 2 in, 2 out]
          }
          frame True {
            w374 = 0 ("Top Row")
            n247 = property on="CheckList" class="LstBox (strict)"() -> ("Number of Rows"=w376:u32)  [unwired: 2 in, 2 out]
            n248 = Initialize Array(0, w376) -> (w375:i32[])
            n249 = property on="CheckList" class="LstBox (strict)"("Top Row"=w374, "Value"=w374, "Item Symbols"=w375) -> ()  [unwired: 2 in, 2 out]
          }
        }
      }
      event "CheckList": Key Down {
        # "Update symbols on the listbox\nLeft and right keys check and uncheck"
        n250 = event-data() -> ("VKey"=w380:T21)  [unwired: 1 in]
        n251 = case shown="\"Left\", \"Right\"" w380 {
          selector: w380 -> [w385 _]
          tunnel: eventvkey."Left" ("VKey") -> [w383 _]
          frame "Left", "Right" {
            n252 = Equal?(x=w383, y=w385) -> (x = y?=w384:bool)
            n253 = Select(t=0, s=w384, f=1) -> (s? t:f=w386:i32)
            n254 = property on="CheckList" class="LstBox (strict)"() -> ("Item Symbols"=w389:i32[])  [unwired: 2 in, 2 out]
            n255 = Replace Array Subset(array=w389, new element=w386, index="CheckList") -> (w388:i32[])
            n256 = property on="CheckList" class="LstBox (strict)"("Item Symbols"=w388) -> ()  [unwired: 2 in, 2 out]
          }
          frame Default {
          }
        }
      }
      event "Motor.Enable": Value Change {
        # "When the test mode otor enable helper is set, update that\ntree row item's value"
        n257 = event-data() -> ("NewVal"=w395:bool)  [unwired: 1 in]
        n258 = Unbundle("Motor") -> ("Value"=w394:dbl)  [unwired: 1 out]
        n259 = Select(t=w394, s=w395, f=0.0) -> (s? t:f=w392:dbl)
        n260 = call <vilib>:"NT Write Number.vi"("Numeric"=w392, "Name"=w391) -> ()  [unwired: 9 in, 1 out]
      }
      event "Test Slider": Value Change {
        # "When the test mode slider helper is set, update that\ntree row item's value"
        n261 = event-data() -> ("NewVal"=w398:dbl)  [unwired: 1 in]
        n262 = call <vilib>:"NT Write Number.vi"("Numeric"=w398, "Name"=w399) -> ()  [unwired: 9 in, 1 out]
      }
      event "On/Off": Value Change {
        # "When the test mode on/off helper value is set, update that\ntree row item's value"
        n263 = event-data() -> ("NewVal"=w403:bool)  [unwired: 1 in]
        n264 = Boolean To (0,1)(Boolean=w403) -> (0, 1=w402:i16)
        n265 = call <vilib>:"NT Write Number.vi"("Numeric"=w402, "Name"=w401) -> ()  [unwired: 9 in, 1 out]
      }
      event "Rev/Fwd": Value Change {
        # "When the test mode helper value for relays is set, update that\ntree row item's value"
        n266 = event-data() -> ("NewVal.Forward"=w411:bool, "NewVal.Reverse"=w410:bool)  [unwired: 1 in]
        n267 = Boolean To (0,1)(Boolean=w411) -> (0, 1=w407:i16)
        n268 = Boolean To (0,1)(Boolean=w410) -> (0, 1=w409:i16)
        n269 = Negate(x=w409) -> (-x=w408:i16)
        n270 = Add(x=w407, y=w408) -> (x+y=w406:i16)
        n271 = call <vilib>:"NT Write Number.vi"("Numeric"=w406, "Name"=w405) -> ()  [unwired: 9 in, 1 out]
      }
      event "Test Ring": Value Change {
        # "When a test mode helper value is selected from the ring,\nset the tree item's variable to the string value"
        n272 = event-data() -> ("NewVal"=w415:u16)  [unwired: 1 in]
        n273 = property on="Test Ring" class="Ring (strict)"() -> ("Strings []"=w416:string[])  [unwired: 2 in, 2 out]
        n274 = Index Array(array=w416, index=w415) -> (element=w414:string)
        n275 = call <vilib>:"NT Write String.vi"("String"=w414, "Name"=w413) -> ()  [unwired: 9 in, 1 out]
      }
      event "Rec Mode": Value Change {
        # "Update globals for recording mode and path to read log from.\nClear when logging and let NetworkTables set path for vision to\nuse."
        n276 = event-data() -> ("NewVal"=w427:enum32{"Stop", "Record", "Playback"})  [unwired: 1 in]
        n277 = global write "WPI_DashboardLogging Global.vi" "Logging Filename"(path "") -> ()
        n278 = global write "WPI_DashboardLogging Global.vi" "Recording"(w427) -> ()
        n279 = case shown="\"Playback\"" w427 {
          tunnel: w426 -> [_ w429 w438]
          tunnel: [_ _ w437] -> w424
          tunnel: [_ _ w436] -> _
          tunnel: w422 -> [_ _ w434]
          tunnel: cluster{i32, i32} {-250, 170} -> [_ _ w433]
          tunnel: [_ _ T22 {"Image Size"=TRUE, "Image Type"=TRUE, "Pixel Value"=TRUE, "ROI Information"=TRUE, "Zoom Factor"=FALSE} ("Image Information Shown:All Elements")] -> w417
          tunnel: [_ _ TRUE ("Zoom Factor")] -> w418
          tunnel: w420 -> [_ _ w430]
          frame Default {
          }
          frame "Stop", "Record" {
            # "Place Window too"
            n280 = invoke class="VI" method="FP.Close"(reference=w429) -> (reference out=w428:refnum<vi>)  [unwired: 2 in, 2 out]
            n281 = invoke class="VI" method="Abort VI"(reference=w428) -> ()  [unwired: 2 in, 3 out]
          }
          frame "Playback" {
            n282 = call "Open Playback Panel.vi"("Offset"=w433, "DB VI Ref"=w434, "Playback in"=w438) -> ("Playback out"=w435:refnum<vi>)  [unwired: 8 in]
            n283 = register-events(w435, w430) -> (reference out=w437:refnum<event-registration>, error out=w436:errorcluster)  [unwired: 2 in]
          }
        }
        n284 = property on="Camera Image Right" class="ImageControl"("Image Information Shown"=w417, "Image Information Visible"=w418) -> ()  [unwired: 2 in, 2 out]
        n285 = property on="Camera Image" class="ImageControl"("Image Information Shown"=w417, "Image Information Visible"=w418) -> ()  [unwired: 2 in, 2 out]
        n286 = call <vilib>:"WPI_DashboardNT Log FieldName Cache.vi"("Operation"=enum16{"Lookup/Add", "Index", "Clear"}."Clear") -> ()  [unwired: 8 in, 3 out]
      }
      event Panel Close {
        w440 = enum32{"Stop", "Record", "Playback"}."Stop" ("Rec Mode")
        # "Playback window has been closed, abort"
        n287 = event-data() -> ()  [unwired: 1 in, 4 out]
        n288 = local write "Rec Mode"(w440) -> ()
        n289 = global write "WPI_DashboardLogging Global.vi" "Recording"(w440) -> ()
      }
      event Panel Close {
        # "Abort playback window and ourself"
        n290 = event-data() -> ()  [unwired: 1 in, 4 out]
        n291 = invoke class="VI" method="FP.Close"(reference=w444) -> (reference out=w443:refnum<vi>)  [unwired: 2 in, 2 out]
        n292 = invoke class="VI" method="Abort VI"(reference=w443) -> (error out=w442:errorcluster)  [unwired: 2 in, 2 out]
        n293 = invoke class="VI" method="Abort VI"(error in=w442) -> ()  [unwired: 2 in, 3 out]
      }
      event User Event {
        n294 = event-data() -> ("IDs"=w451:cluster{"RPC field ID":u16, "Unique ID":u16}, "String"=w450:string)  [unwired: 1 in]
        n295 = Bundle("IDs"=w451, "String"=w450) -> (w449:T10)  [unwired: 1 in]
        n296 = call <vilib>:"Retrieve RPC Response.vi"("RPC Response"=w449) -> ("Output"=w447:string[][])  [unwired: 10 in]
        n297 = Build Array (concatenate)(w445, w447) -> (w446:string[][])
        n298 = local write "Command Params"(w446) -> ()
        n299 = local write "Cmd Status"("" ("Cmd Status")) -> ()
      }
      event "Tree": Double Click {
        n300 = event-data() -> ("PlatMods"=w457:T25, "Tag"=w454:string)  [unwired: 1 in]
        n301 = Unbundle(w457) -> ("Shift"=w456:bool)  [unwired: 4 out]
        n302 = String Subset(string=w454, length (rest)=1 ("length (rest)")) -> (substring=w453:string)  [unwired: 1 in]
        n303 = Not(x=w456) -> (.not. x?=w455:bool)
        n304 = case shown="\"/\"" w453 {
          tunnel: w454 -> [_ w460]
          tunnel: w455 -> [_ w459]
          frame Default {
          }
          frame "/" {
            n305 = call <vilib>:"NT Update Persistence.vi"("Persistence"=w459, "Name"=w460) -> ()  [unwired: 9 in, 1 out]
          }
        }
      }
    }
  }
  n306 = while {
    tunnel: w36 -> [w462]
    i -> [w465]
    stop <- FALSE stop-if-true
    n307 = Wait (ms)(milliseconds to wait=u32 100) -> ()  [unwired: 1 out]
    n308 = case shown="\"Playback\"" "Rec Mode" {
      tunnel: w465 -> [_ _ w480]
      tunnel: [u32 2829099 ("Base Color") u32 11141120 ("Target Color") w469] -> w461
      frame "Stop", Default {
        # "Reset the color, extra updates don't cost much"
      }
      frame "Record" {
      }
      frame "Playback" {
        # "Playback"
        n309 = Quotient & Remainder(x=w480, y=u32 50 ("milliseconds to wait")) -> (x-y*floor(x/y)=w476:u32)  [unwired: 1 out]
        n310 = Divide(x=w476, y=u32 50 ("milliseconds to wait")) -> (x/y=w473:dbl)
        n311 = Multiply(x=6.283185307179586, y=w473) -> (x*y=w478:dbl)
        n312 = Sine(x=w478) -> (sin(x)=w477:dbl)
        n313 = Absolute Value(x=w477) -> (abs(x)=w470:dbl)
        n314 = call "Interpolate RGB Color.vi"("Proportion"=w470, "Target Color"=u32 30976, "Base Color"=u32 2829099) -> ("Result Color"=w469:u32)  [unwired: 8 in]
      }
    }
    n315 = property class="Pane"(reference=w462, "PaneColor"=w461) -> ()  [unwired: 1 in, 2 out]
  }
  n316 = local write "Dashboard Tab"(T3."Drive" ("Dashboard Tab")) -> ()
  n317 = property on="On/Off" class="Bool (strict)"("Visible"=w25) -> ()  [unwired: 2 in, 2 out]
  n318 = property on="Motor" class="Clust (strict)"("Visible"=w25) -> ()  [unwired: 2 in, 2 out]
  n319 = property on="Progress" class="Clust (strict)"("Visible"=w25) -> ()  [unwired: 2 in, 2 out]
  n320 = property on="Test Ring" class="Ring (strict)"("Visible"=w25) -> ()  [unwired: 2 in, 2 out]
  n321 = property on="Rev/Fwd" class="Clust (strict)"("Visible"=w25) -> ()  [unwired: 2 in, 2 out]
  n322 = while {
    stop <- FALSE stop-if-true
    n323 = call-poly <vilib>:"NT Read Value.vi"("Name"="DriveSensorData") -> ("Variant"=w495:variant)  [unwired: 9 in, 1 out]
    n324 = call-poly <vilib>:"NT Read Value.vi"("Name"="AutoFiles") -> ("String Array"=→"AutoFilesOnRobot":string[])  [unwired: 9 in, 1 out]
    n325 = Variant To Data(type=T1 {"LeftDistance"=0.0, "RightDistance"=0.0, "LeftVelocity"=0.0, "RightVelocity"=0.0, "Angle"=0.0, "Location"={0.0, 0.0}} ("SensorData"), Variant=w495) -> (data=→"DriveSensorData":T1)  [unwired: 1 in, 1 out]
    n326 = To Upper Case(1:"AutoFileName (No .txt)") -> (0:w481:string)
    n327 = call-poly <vilib>:"NT Write Value.vi"("String"=w481, "Name"="AutoFile") -> ()  [unwired: 9 in, 1 out]
    n328 = call-poly <vilib>:"NT Write Value.vi"("Numeric"="WaitAtStartOfAuto (Seconds)", "Name"="AutoDelay") -> ()  [unwired: 9 in, 1 out]
    n329 = call-poly <vilib>:"NT Write Value.vi"("Numeric"="StartingPosition", "Name"="StartingPosition") -> ()  [unwired: 9 in, 1 out]
    n330 = Wait (ms)(milliseconds to wait=u32 100) -> ()  [unwired: 1 out]
  }
  n331 = while {
    tunnel: u16 1741 ("timeout ms (25000)") -> [w497]
    stop <- FALSE stop-if-true
    n332 = TCP Create Listener(10:w497) -> (0:w496:errorcluster, 3:w498:refnum<k5>)  [unwired: 4 in, 1 out]
    n333 = case shown="No Error" w496 {
      selector: w496 -> [w500 _]
      tunnel: w498 -> [w501 _]
      frame No Error {
        n334 = while {
          tunnel: w501 -> [w504]
          tunnel: w500 -> [w503]
          stop <- FALSE stop-if-true
          n335 = TCP Wait On Listener(8:w503, 11:w504) -> (0:w505:errorcluster, 4:w506:refnum<k5>)  [unwired: 2 in, 3 out]
          n336 = local write "TCP"(w506) -> ()
          n337 = case shown="No Error" w505 {
            frame No Error {
            }
            frame Error {
              n338 = Wait (ms)(milliseconds to wait=u32 1000) -> ()  [unwired: 1 out]
            }
          }
        }
      }
      frame Error {
        n339 = Wait (ms)(milliseconds to wait=u32 1000) -> ()  [unwired: 1 out]
      }
    }
  }
  n340 = local write "Command Selection"(u16 0 ("milliseconds to wait")) -> ()
  n341 = local write "Command Params"(string[][] [] ("Command Params")) -> ()
  n342 = global write "WPI_DashboardLogging Global.vi" "Recording"(w30) -> ()
  n343 = local write "Rec Mode"(w30) -> ()
  n344 = call <vilib>:"NT Write String.vi"("Name"="Auto Selector") -> ()  [unwired: 10 in, 1 out]
